vi "Login Status (SubVI).vi"() -> (3 "Numeric":i32)   [LabVIEW 2023]
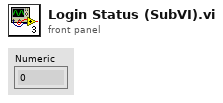
[diagram p1: front panel]
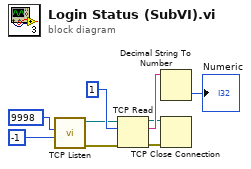
[diagram p0: block diagram]
diagram:
  n1 = call <vilib>:"TCP Listen.vi"("timeout ms (wait forever: -1)"=-1, "port"=u16 9998) -> ("error out"=w1:errorcluster, "connection ID"=w2:refnum<k5>)  [unwired: 5 in, 3 out]
  n2 = TCP Read(connection ID=w2, bytes to read=1, error in (no error)=w1) -> (connection ID out=w5:refnum<k5>, data out=w7:string, error out=w6:errorcluster)  [unwired: 2 in]
  n3 = Decimal String To Number(string=w7) -> (number=→"Numeric":i32)  [unwired: 2 in, 1 out]
  n4 = TCP Close Connection(connection ID=w5, error in (no error)=w6) -> ()  [unwired: 1 in, 2 out]
